vi "Launch Module.vi"(8 "error in":errorcluster) -> (0 "error out":errorcluster)   [LabVIEW 2021, in "Host Interpreter.lvlib"]
uses:
  Host Interpreter.lvlib
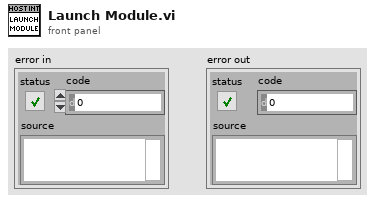
[diagram p1: front panel]
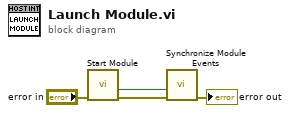
[diagram p0: block diagram]
diagram:
  n1 = call "Start Module.vi"("error in"="error in") -> ("error out"=w3:errorcluster, "Wait for Event Sync?"=w4:bool)  [unwired: 6 in, 3 out]
  n2 = call "Synchronize Module Events.vi"("error in"=w3, "Wait for Event Sync?"=w4) -> ("error out"=→"error out":errorcluster)  [unwired: 9 in]
